vi "MessungHB_Periode.vi"(7 "Faktor 1":dbl=1.0, 8 "Error_in":errorcluster, 9 "Faktor2 (1)":dbl=1.0, 10 "Anzahl der Messpunkte":i32=6000, 11 "VISA Name OZ in(OZ)":refnum<visa-resource-name>="USB0::0x0957::0x179B::MY54313507::INSTR") -> (0 "Error_out":errorcluster, 1 "H-Messdaten einer periode":dbl[](array[numeric]), 2 "B-Messdaten einer periode":dbl[](array[numeric]), 3 "VISA Name OZ out(OZ)":refnum<visa-resource-name>="USB0::0x0957::0x179B::MY54313507::INSTR")   [LabVIEW 2016]
doc: "Dieses VI führt eine Skalierung und Messung von Channel 1 durch. Die gemessenen Werte werden auf eine Periode limitiert. Das gleiche geschieht mit Channel 2.\n\nAm Ausgang des VI's können die H & B Array abgegriffen werden."
uses:
  controls/Oszi_KanalInfo.ctl
panel:
  out "Anzahl Messwerte B":i32
  out "Anzahl Messwerte H":i32
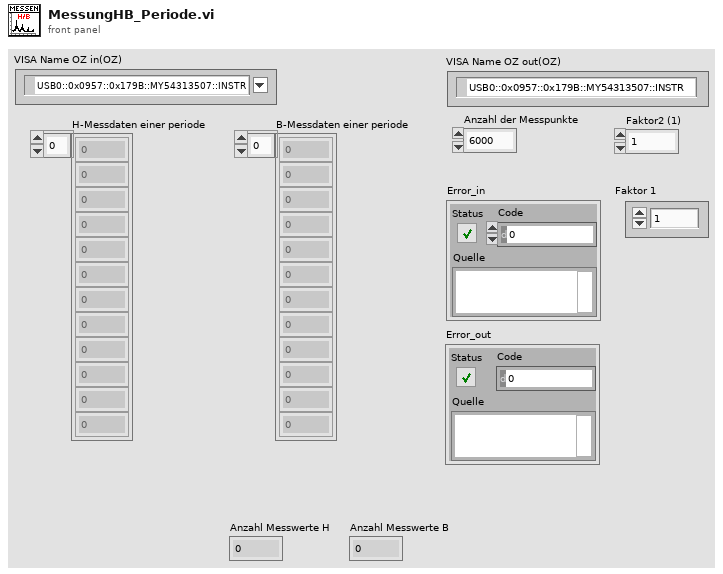
[diagram p1: front panel]
types:
  T1 = typedef "Oszi_KanalInfo.ctl" = dbl
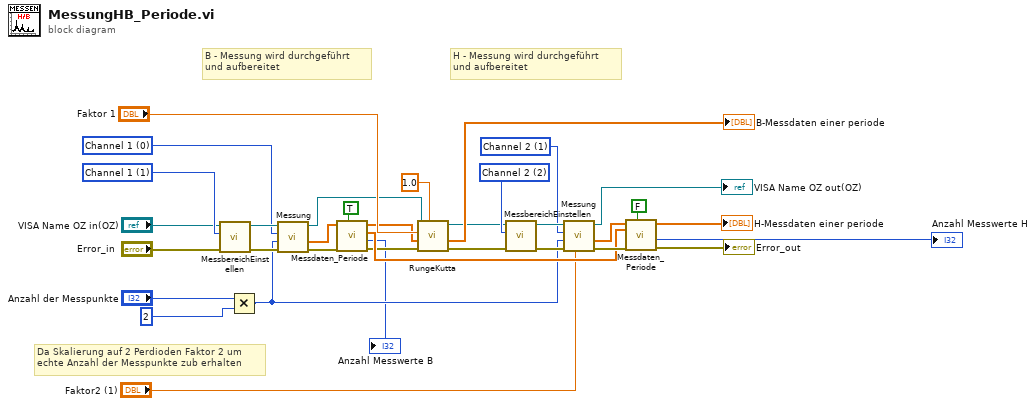
[diagram p0: block diagram]
diagram:
  w27 = 1 items=["Channel 1"=1, "Channel 2"=2, "Channel 3"=3, "Channel 4"=4] ("Channel Name (1: Channel 1)")
  w28 = 0 items=["Channel 1"=0, "Channel 2"=1, "Channel 3"=2, "Channel 4"=3, "Waveform Memory 1"=5, "Waveform Memory 2"=6, "Serial Bus 1"=7, "Serial Bus 2"=8, "Digital Bus Low"=9, "Digital Bus High "=10, "Digital Bus 1"=11, "Digital Bus 2"=12, "Function 1"=32, "Function 2"=33, "Function 3"=34, "Function 4"=35, "Math 1"=36, "Math 2"=37, "Math 3"=38, "Math 4"=39] ("Source Channel (0: Channel 1)")
  w29 = 2 items=["Channel 1"=1, "Channel 2"=2, "Channel 3"=3, "Channel 4"=4] ("Channel Name (1: Channel 1)")
  w30 = 1 items=["Channel 1"=0, "Channel 2"=1, "Channel 3"=2, "Channel 4"=3, "Waveform Memory 1"=5, "Waveform Memory 2"=6, "Serial Bus 1"=7, "Serial Bus 2"=8, "Digital Bus Low"=9, "Digital Bus High "=10, "Digital Bus 1"=11, "Digital Bus 2"=12, "Function 1"=32, "Function 2"=33, "Function 3"=34, "Function 4"=35, "Math 1"=36, "Math 2"=37, "Math 3"=38, "Math 4"=39] ("Source Channel (0: Channel 1)")
  # "H - Messung wird durchgeführt\nund aufbereitet"
  # "B - Messung wird durchgeführt\nund aufbereitet"
  # "Da Skalierung auf 2 Perdioden Faktor 2 um \nechte Anzahl der Messpunkte zub erhalten"
  n1 = call "MessbereichEinstellen.vi"("Error_in"="Error_in", "Channel Name (1: Channel 1)"=w27, "VISA Name OZ in(OZ)"="VISA Name OZ in(OZ)") -> ("Error_out"=w34:errorcluster, "VISA Name OZ out"=w33:refnum<visa-resource-name>)  [unwired: 7 in]
  n2 = Multiply(x="Anzahl der Messpunkte", y=2) -> (x*y=w21:i32)
  n3 = call "Messung.vi"("error in"=w34, "Points (6000)"=w21, "Source Channel (0: Channel 1)"=w28, "VISA resource name(OZ)"=w33) -> ("error out"=w26:errorcluster, "Messdaten"=w6:dbl[], "VISA resource name out"=w7:refnum<visa-resource-name>)  [unwired: 4 in, 1 out]
  n4 = call "Messdaten_Periode.vi"("Quelle Indices (Erzeugen=1, Extern=0)"=TRUE ("Auswertung"), "error in"=w26, "Messdaten_Eingang(1-D)"=w6) -> ("error out"=w13:errorcluster, "Anzahl Messwerte"=→"Anzahl Messwerte B":i32, "Indices_der_Schwellwerte"=w22:dbl[], "Messdaten_einer_periode"=w4:dbl[])  [unwired: 3 in, 2 out]
  n5 = call "RungeKutta.vi"("Oszi-Channel (1)"=T1 1.0, "error in (no error)"=w13, "Messdaten In"=w4, "faktor1"="Faktor 1", "VISA Name OZ In (OZ)"=w7) -> ("error out"=w12:errorcluster, "Output Array B Out"=→"B-Messdaten einer periode":dbl[], "VISA Name OZ Out"=w11:refnum<visa-resource-name>)  [unwired: 4 in]
  n6 = call "MessbereichEinstellen.vi"("Error_in"=w12, "Channel Name (1: Channel 1)"=w29, "VISA Name OZ in(OZ)"=w11) -> ("Error_out"=w31:errorcluster, "VISA Name OZ out"=w32:refnum<visa-resource-name>)  [unwired: 7 in]
  n7 = call "Messung.vi"("Faktor2 (1)"="Faktor2 (1)", "error in"=w31, "Points (6000)"=w21, "Source Channel (0: Channel 1)"=w30, "VISA resource name(OZ)"=w32) -> ("error out"=w25:errorcluster, "Messdaten"=w5:dbl[], "VISA resource name out"=→"VISA Name OZ out(OZ)":refnum<visa-resource-name>)  [unwired: 3 in, 1 out]
  n8 = call "Messdaten_Periode.vi"("Quelle Indices (Erzeugen=1, Extern=0)"=FALSE ("Auswertung"), "error in"=w25, "Messdaten_Indices_Extern"=w22, "Messdaten_Eingang(1-D)"=w5) -> ("error out"=→"Error_out":errorcluster, "Anzahl Messwerte"=→"Anzahl Messwerte H":i32, "Messdaten_einer_periode"=→"H-Messdaten einer periode":dbl[])  [unwired: 2 in, 3 out]
